vi "Launcher_Wheel_v4.vi"() -> ()   [LabVIEW 2011]
uses:
  StateMachineType.ctl
  BasketType.ctl
  FormulaChoose.ctl
  Robot Global Data.vi
  <vilib>/addons/control/pid/pid.llb/PID (DBL).vi
  <vilib>/addons/control/pid/NI_PID_pid.lvlib
panel:
  out "Encoder R":dbl
  out "Encoder L":dbl
  in  "PID R":T1={"proportional gain (Kc)"=0.0008, "integral time (Ti, min)"=0.010000000000000009, "derivative time (Td, min)"=0.0} {"derivative time (Td, min)" step=0.01 format="%.2f"; "integral time (Ti, min)" step=0.01 format="%.2f"; "proportional gain (Kc)" step=0.0001 format="%.4f"}
  in  "Output R":cluster{"output high":dbl, "output low":dbl}={"output high"=1.0, "output low"=0.0} {"output low" step=0.1 format="%.2f"; "output high" step=0.1 format="%.2f"}
  in  "Output L":cluster{"output high":dbl, "output low":dbl}={"output high"=1.0, "output low"=0.0} {"output low" step=0.1 format="%.2f"; "output high" step=0.1 format="%.2f"}
  in  "PID L":T1={"proportional gain (Kc)"=0.0008, "integral time (Ti, min)"=0.01, "derivative time (Td, min)"=0.0} {"derivative time (Td, min)" step=0.01 format="%.2f"; "integral time (Ti, min)" step=0.01 format="%.2f"; "proportional gain (Kc)" step=0.0001 format="%.4f"}
  out "R Status":bool
  out "L Status":bool
  in  "Encoder Control L (PC)":dbl(slide) step=100.0 scale=0.0..1400.0
  in  "Encoder Control R (PC)":dbl(slide) step=100.0 scale=0.0..1400.0
  in  "Set RPM (PC)":dbl(slide) step=100.0 scale=0.0..1400.0
  in  "Gamepad Adjust (PC)":dbl(slide) step=0.1 scale=1.0..-1.0
  in  "Autonomous (PC)":bool
  in  "Which Formula?":T2
  in  "Basket (PC)":T3=enum."Top"
  in  "Direct Motor Control":bool
  out "Calculation Failed":bool
  in  "Distance (PC)":dbl
  out "Motor R Input":dbl
  out "Motor L Input":dbl
  out "Loop Status":T4
  in  "RunLauncher (PC)":bool
  # "For testing on computer only"
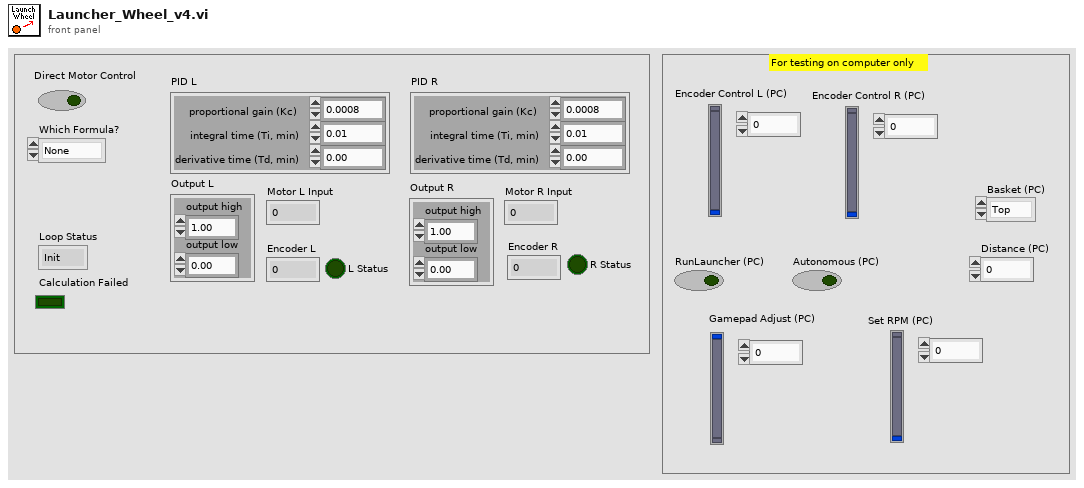
[diagram p1: front panel]
types:
  T1 = cluster{"proportional gain (Kc)":dbl, "integral time (Ti, min)":dbl, "derivative time (Td, min)":dbl}
  T2 = typedef "FormulaChoose.ctl" = enum16{"None", "Brian", "Jeremy", "Steven", "Data Based"}
  T3 = typedef "BasketType.ctl" = enum16{"Left", "Bottom", "Right", "Top"}
  T4 = typedef "StateMachineType.ctl" = enum16{"Init", "Idle", "Start", "Do", "Stop"}
  T5 = typedef "WPI_MotorControlDeviceRef.ctl" = cluster{"DeviceStatus":errorcluster, "Type":enum16{"PWM", "CAN"}, "PWM":cluster{"Digital Module":T6, "PWM Channel":T7, "DeadBand":T8}, "CAN":cluster{"Device Number":u8, "Control Mode":T9, "Semaphore":T10, "Max Vout":dbl}, "Invert":bool, "TransformRef":T11, "InvTransformRef":T11}
  T6 = typedef "FPGA_TypedefDigitalModule.ctl" = enum16{"Digital Module 1", "Digital Module 2"}
  T7 = typedef "FPGA_DIOPWMChannel.ctl" = enum8{"PWM 1", "PWM 2", "PWM 3", "PWM 4", "PWM 5", "PWM 6", "PWM 7", "PWM 8", "PWM 9", "PWM 10", "Invalid"}
  T8 = typedef "WPI_PWMDeadband.ctl" = cluster{"Name":string, "maxPositivePwm":i32, "minPositivePwm":i32, "centerPwm":i32, "maxNegativePwm":i32, "minNegativePwm":i32, "angularRange":u16}
  T9 = typedef "WPI_CANJaguar_ControlMode.ctl" = enum8{"Percent VBus", "Current", "Speed", "Position", "Voltage"}
  T10 = typedef "Semaphore RefNum" = refnum<k1>
  T11 = typedef "WPI_PWMTransform_ConPane.ctl" = refnum<vi>
  T12 = typedef "WPI_CounterDevRef.ctl" = cluster{"DevStatus":errorcluster, "CntIndex":T13}
  T13 = typedef "FPGA_CounterCtrSystemIndex.ctl" = enum8{"Ctr 0", "Ctr 1", "Ctr 2", "Ctr 3", "Ctr 4", "Ctr 5", "Ctr 6", "Ctr 7", "Invalid"}
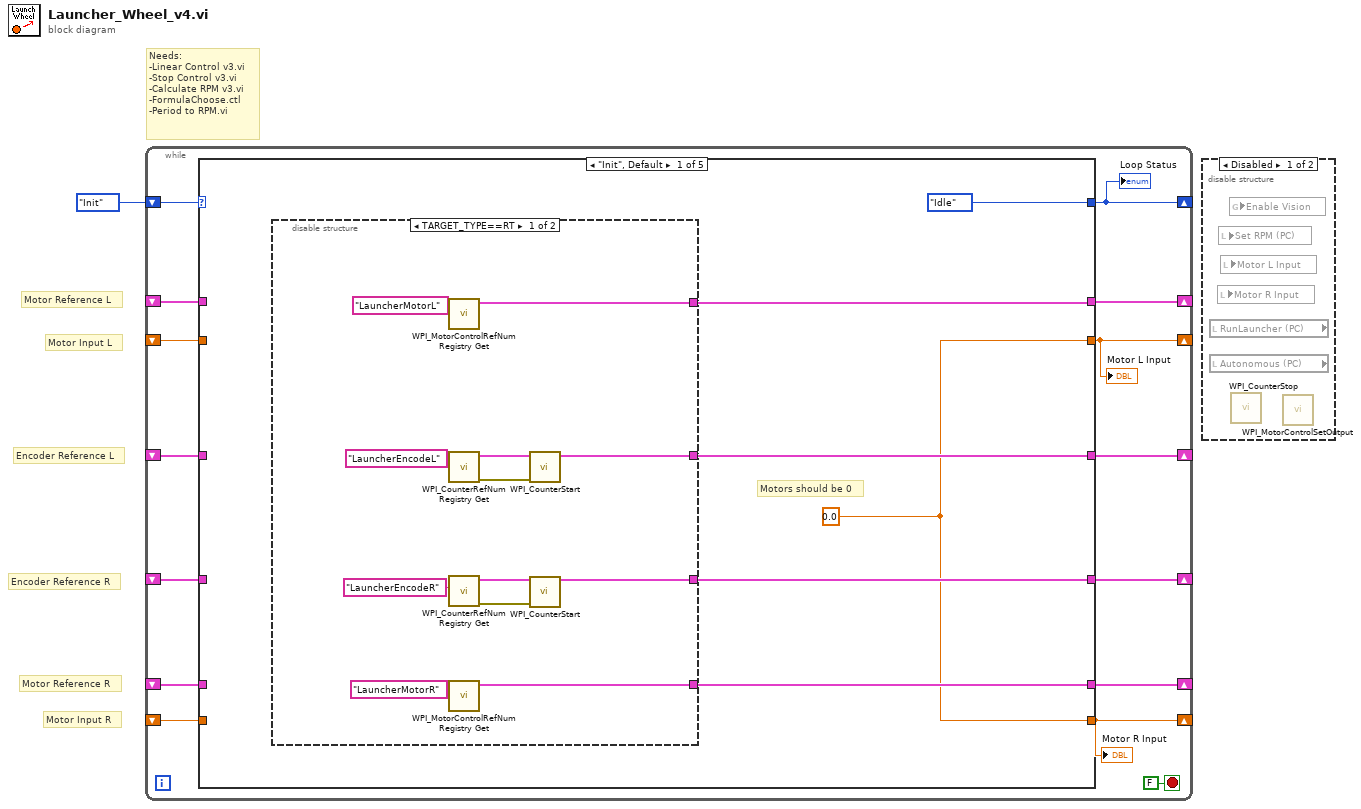
[diagram p0: block diagram]
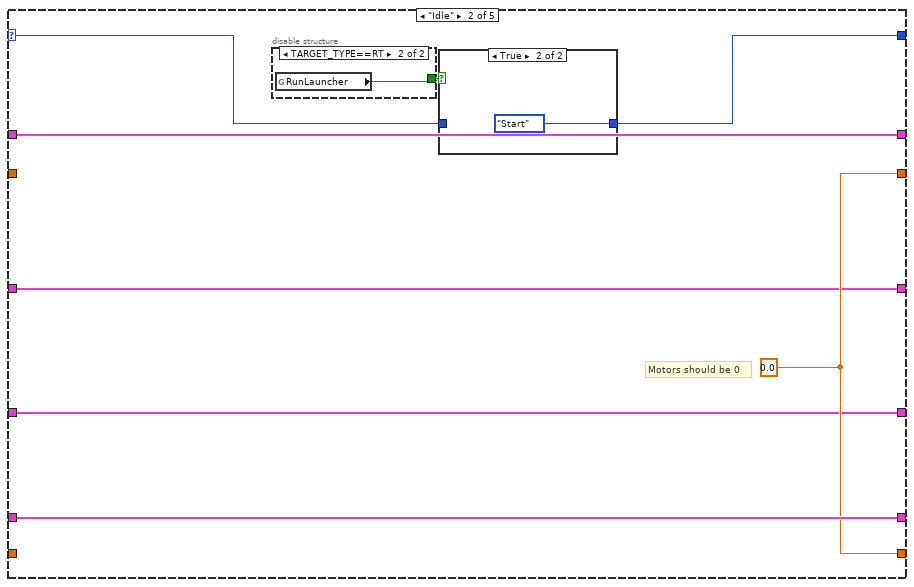
[diagram p4: hidden frame]
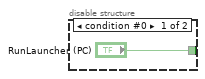
[diagram p5: hidden frame]
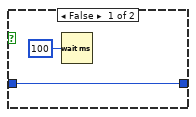
[diagram p6: hidden frame]
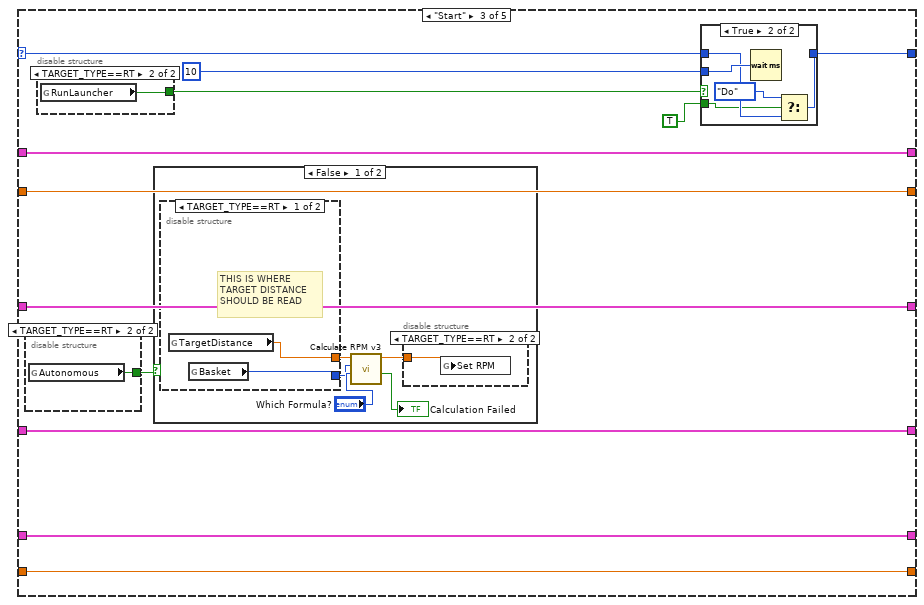
[diagram p7: hidden frame]
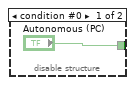
[diagram p8: hidden frame]
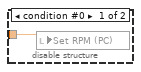
[diagram p9: hidden frame]
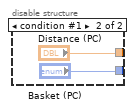
[diagram p10: hidden frame]
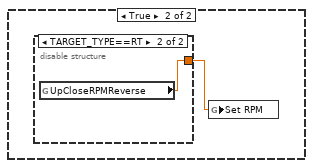
[diagram p11: hidden frame]
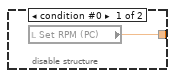
[diagram p12: hidden frame]
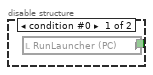
[diagram p13: hidden frame]
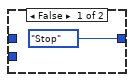
[diagram p14: hidden frame]
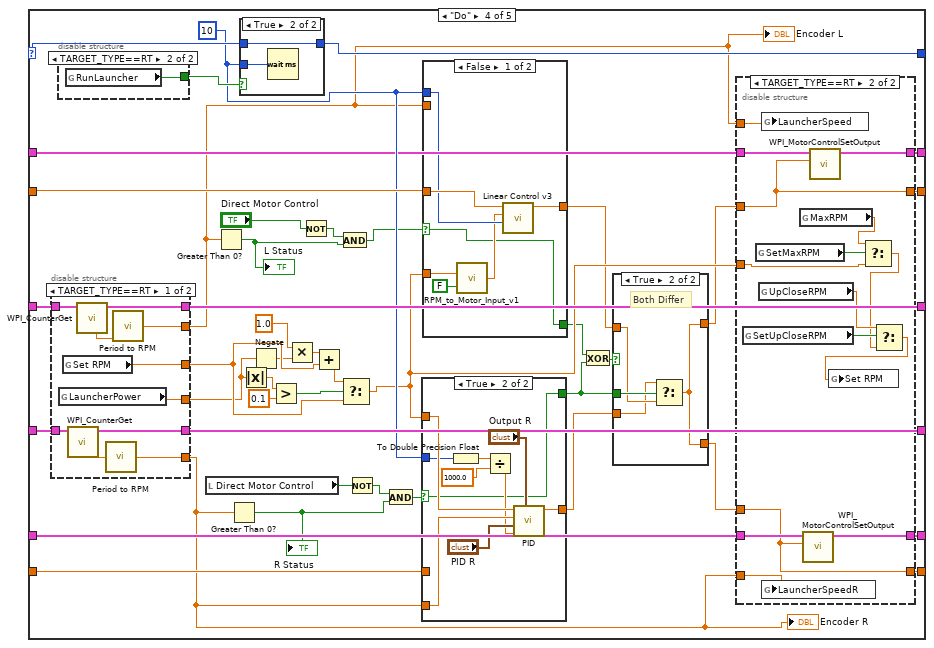
[diagram p15: hidden frame]
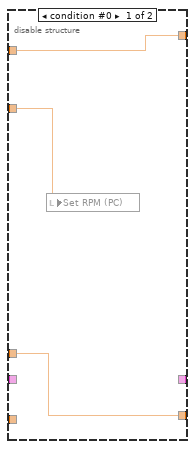
[diagram p17: hidden frame]
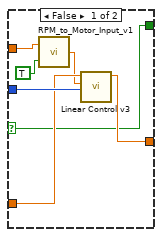
[diagram p18: hidden frame]
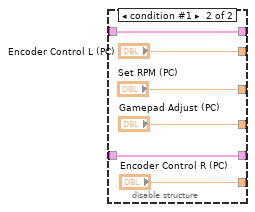
[diagram p19: hidden frame]
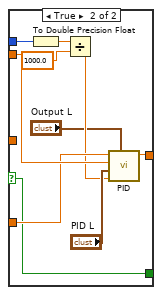
[diagram p20: hidden frame]
diagram:
  # "Needs:\n-Linear Control v3.vi\n-Stop Control v3.vi\n-Calculate RPM v3.vi\n-FormulaChoose.ctl\n-Period to RPM.vi"
  # "Motor Input R"
  # "Encoder Reference R"
  # "Motor Reference R"
  # "Encoder Reference L"
  # "Motor Reference L"
  # "Motor Input L"
  n1 = while {
    shift-right: [w2] -> _
    shift-left: StateMachineType."Init" ("Enum") -> [w15]
    shift-right: [w13] -> _
    shift-left: _ -> [w11]
    shift-right: [w14] -> _
    shift-left: _ -> [w12]
    shift-right: [w3] -> _
    shift-left: _ -> [w9]
    shift-right: [w4] -> _
    shift-left: _ -> [w10]
    shift-right: [w8] -> _
    shift-left: _ -> [w6]
    shift-right: [w7] -> _
    shift-left: _ -> [w5]
    stop <- FALSE stop-if-true
    n2 = case shown="\"Init\", Default" w15 {
      selector: w15 -> [_ w36 w57 w125 w215]
      tunnel: [StateMachineType."Idle" ("Enum") w35 w53 w124 w216] -> w2
      tunnel: [w21 w42 w51 w112 w214] -> w14
      tunnel: [w18 w41 w50 w111 w213] -> w13
      tunnel: w12 -> [_ w42 w51 w114 w211]
      tunnel: w11 -> [_ w41 w50 w113 w212]
      tunnel: [w17 w39 w48 w110 w209] -> w3
      tunnel: [w17 w39 w49 w109 w210] -> w4
      tunnel: w10 -> [_ _ w49 w117 w221]
      tunnel: w9 -> [_ _ w48 w116 w220]
      tunnel: [w19 w38 w56 w121 w208] -> w8
      tunnel: [w20 w37 w55 w120 w207] -> w7
      tunnel: w6 -> [_ w38 w56 w123 w208]
      tunnel: w5 -> [_ w37 w55 w122 w207]
      frame "Init", Default {
        w17 = 0.0
        # "Motors should be 0"
        n3 = disable-structure shown="TARGET_TYPE==RT" {
          disable-tunnel: [w32 _] -> w21
          disable-tunnel: [w31 _] -> w18
          disable-tunnel: [w27 _] -> w19
          disable-tunnel: [w28 _] -> w20
          frame condition #0 (active) {
            n4 = call <vilib>:"WPI_MotorControlRefNum Registry Get.vi"("refnum name"="LauncherMotorL") -> ("MotorControlDevRef"=w32:T5)  [unwired: 9 in, 1 out]
            n5 = call <vilib>:"WPI_CounterRefNum Registry Get.vi"("refnum name"="LauncherEncodeL") -> ("error out"=w23:errorcluster, "CounterDevRef"=w26:T12)  [unwired: 9 in]
            n6 = call <vilib>:"WPI_CounterRefNum Registry Get.vi"("refnum name"="LauncherEncodeR") -> ("error out"=w24:errorcluster, "CounterDevRef"=w25:T12)  [unwired: 9 in]
            n7 = call <vilib>:"WPI_MotorControlRefNum Registry Get.vi"("refnum name"="LauncherMotorR") -> ("MotorControlDevRef"=w31:T5)  [unwired: 9 in, 1 out]
            n8 = call <vilib>:"WPI_CounterStart.vi"("error in (no error)"=w23, "CounterDevRef in"=w26) -> ("CounterDevRef out"=w27:T12)  [unwired: 8 in, 1 out]
            n9 = call <vilib>:"WPI_CounterStart.vi"("error in (no error)"=w24, "CounterDevRef in"=w25) -> ("CounterDevRef out"=w28:T12)  [unwired: 8 in, 1 out]
          }
          frame condition #1 {
          }
        }
      }
      frame "Idle" {
        w39 = 0.0 ("New Motor Input")
        # "Motors should be 0"
        n10 = disable-structure shown="TARGET_TYPE==RT" {
          disable-tunnel: ["RunLauncher (PC)" w44] -> w40
          frame condition #0 {
          }
          frame condition #1 (active) {
            n11 = global read "Robot Global Data.vi" "RunLauncher"() -> (w44:bool)
          }
        }
        n12 = case shown="True" w40 {
          tunnel: w36 -> [w45 _]
          tunnel: [w45 StateMachineType."Start" ("Enum")] -> w35
          frame False {
            n13 = Wait (ms)(milliseconds to wait=u32 100) -> ()  [unwired: 1 out]
          }
          frame True {
          }
        }
      }
      frame "Start" {
        n14 = disable-structure shown="TARGET_TYPE==RT" {
          disable-tunnel: ["Autonomous (PC)" w61] -> w54
          frame condition #0 {
          }
          frame condition #1 (active) {
            n15 = global read "Robot Global Data.vi" "Autonomous"() -> (w61:bool)
          }
        }
        n16 = disable-structure shown="TARGET_TYPE==RT" {
          disable-tunnel: [w76 w77] -> w58
          frame condition #0 {
            n17 = local read "RunLauncher (PC)"() -> (w76:bool)
          }
          frame condition #1 (active) {
            n18 = global read "Robot Global Data.vi" "RunLauncher"() -> (w77:bool)
          }
        }
        n19 = case shown="False" w54 {
          frame False {
            n20 = disable-structure shown="TARGET_TYPE==RT" {
              disable-tunnel: [w69 "Distance (PC)"] -> w63
              disable-tunnel: [w70 "Basket (PC)"] -> w62
              frame condition #0 (active) {
                # "THIS IS WHERE\nTARGET DISTANCE\nSHOULD BE READ"
                n21 = global read "Robot Global Data.vi" "TargetDistance"() -> (w69:dbl)
                n22 = global read "Robot Global Data.vi" "Basket"() -> (w70:T3)
              }
              frame condition #1 {
              }
            }
            n23 = call "Calculate RPM v3.vi"("Which Formula"="Which Formula?", "Basket"=w62, "Distance to Target (feet)"=w63) -> ("Calculation Failed"=→"Calculation Failed":bool, "RPM"=w64:dbl)  [unwired: 6 in, 1 out]
            n24 = disable-structure shown="TARGET_TYPE==RT" {
              disable-tunnel: w64 -> [w67 w68]
              frame condition #0 {
                n25 = local write "Set RPM (PC)"(w67) -> ()
              }
              frame condition #1 (active) {
                n26 = global write "Robot Global Data.vi" "Set RPM"(w68) -> ()
              }
            }
          }
          frame True {
            n27 = disable-structure shown="TARGET_TYPE==RT" {
              disable-tunnel: [w74 w75] -> w73
              frame condition #0 {
                n28 = local read "Set RPM (PC)"() -> (w74:dbl)
              }
              frame condition #1 (active) {
                n29 = global read "Robot Global Data.vi" "UpCloseRPMReverse"() -> (w75:dbl)
              }
            }
            n30 = global write "Robot Global Data.vi" "Set RPM"(w73) -> ()
          }
        }
        n31 = case shown="True" w58 {
          tunnel: u32 10 ("milliseconds to wait") -> [_ w83]
          tunnel: [StateMachineType."Stop" w80] -> w53
          tunnel: w57 -> [_ w82]
          tunnel: TRUE -> [_ w79]
          frame False {
          }
          frame True {
            n32 = Wait (ms)(milliseconds to wait=w83) -> ()  [unwired: 1 out]
            n33 = Select(t=StateMachineType."Do" ("Enum"), s=w79, f=w82) -> (s? t:f=w80:T4)
          }
        }
      }
      frame "Do" {
        w115 = u32 10 ("milliseconds to wait")
        n34 = disable-structure shown="TARGET_TYPE==RT" {
          disable-tunnel: w122 -> [w168 w182]
          disable-tunnel: w123 -> [w177 w183]
          disable-tunnel: [w176 w182] -> w120
          disable-tunnel: [w175 w183] -> w121
          disable-tunnel: [w171 "Encoder Control L (PC)"] -> w107
          disable-tunnel: [w173 "Encoder Control R (PC)"] -> w108
          disable-tunnel: [w170 "Set RPM (PC)"] -> w119
          disable-tunnel: [w169 "Gamepad Adjust (PC)"] -> w118
          frame condition #0 (active) {
            n35 = global read "Robot Global Data.vi" "LauncherPower"() -> (w169:dbl)
            n36 = global read "Robot Global Data.vi" "Set RPM"() -> (w170:dbl)
            n37 = call <vilib>:"WPI_CounterGet.vi"("CounterDevRef in"=w168) -> ("CounterDevRef out"=w176:T12, "Period (sec)"=w174:dbl)  [unwired: 5 in, 4 out]
            n38 = call <vilib>:"WPI_CounterGet.vi"("CounterDevRef in"=w177) -> ("CounterDevRef out"=w175:T12, "Period (sec)"=w172:dbl)  [unwired: 5 in, 4 out]
            n39 = call "Period to RPM.vi"("Period (sec)"=w174) -> ("Numeric Control"=w173:dbl)
            n40 = call "Period to RPM.vi"("Period (sec)"=w172) -> ("Numeric Control"=w171:dbl)
          }
          frame condition #1 {
          }
        }
        "Encoder R" <- w108
        "Encoder L" <- w107
        n41 = disable-structure shown="TARGET_TYPE==RT" {
          disable-tunnel: [w201 w202] -> w126
          frame condition #0 {
            n42 = local read "RunLauncher (PC)"() -> (w201:bool)
          }
          frame condition #1 (active) {
            n43 = global read "Robot Global Data.vi" "RunLauncher"() -> (w202:bool)
          }
        }
        n44 = local read "Direct Motor Control"() -> (w98:bool)
        n45 = Greater Than 0?(x=w107) -> (x > 0?=w93:bool)
        "L Status" <- w93
        n46 = Greater Than 0?(x=w108) -> (x > 0?=w96:bool)
        "R Status" <- w96
        n47 = case shown="True" w126 {
          tunnel: w115 -> [_ w205]
          tunnel: w125 -> [_ w204]
          tunnel: [StateMachineType."Stop" ("Enum") w204] -> w124
          frame False {
          }
          frame True {
            n48 = Wait (ms)(milliseconds to wait=w205) -> ()  [unwired: 1 out]
          }
        }
        n49 = Absolute Value(x=w118) -> (abs(x)=w104:dbl)
        n50 = Negate(x=w118) -> (-x=w103:dbl)
        n51 = Greater?(x=w104, y=0.1) -> (0:w105:bool)
        n52 = Multiply(x=1.0, y=w103) -> (x*y=w101:dbl)
        n53 = Not(x="Direct Motor Control") -> (.not. x?=w94:bool)
        n54 = Add(x=w101, y=w119) -> (x+y=w100:dbl)
        n55 = And(x=w94, y=w93) -> (x .and. y?=w91:bool)
        n56 = Select(t=w100, s=w105, f=w119) -> (s? t:f=w99:dbl)
        n57 = Not(x=w98) -> (.not. x?=w97:bool)
        n58 = And(x=w97, y=w96) -> (x .and. y?=w95:bool)
        n59 = case shown="True" w95 {
          selector: w95 -> [w151 w158]
          tunnel: w116 -> [w156 _]
          tunnel: w99 -> [w153 w165]
          tunnel: w108 -> [_ w164]
          tunnel: w115 -> [w157 w161]
          tunnel: [w155 w159] -> w86
          tunnel: [w151 w158] -> w88
          frame False {
            n60 = call "RPM_to_Motor_Input_v1.vi"("Right Motor?"=TRUE, "RPM"=w153) -> ("Motor Input"=w154:dbl)
            n61 = call "Linear Control v3.vi"("Loop Time (ms)"=w157, "Setpoint"=w154, "Recieved Motor Input"=w156) -> ("New Motor Input"=w155:dbl)  [unwired: 7 in, 1 out]
          }
          frame True {
            n62 = To Double Precision Float(number=w161) -> (double precision float=w163:dbl)
            n63 = Divide(x=w163, y=1000.0) -> (x/y=w160:dbl)
            n64 = call-poly <vilib>:"PID.vi"("output range"="Output R", "dt (s)"=w160, "PID gains"="PID R", "process variable"=w164, "setpoint"=w165) -> ("output"=w159:dbl)  [unwired: 5 in, 1 out]
          }
        }
        n65 = case shown="False" w91 {
          selector: w91 -> [w184 w191]
          tunnel: w117 -> [w190 _]
          tunnel: w99 -> [w186 w199]
          tunnel: w107 -> [_ w200]
          tunnel: w115 -> [w189 w197]
          tunnel: [w188 w192] -> w87
          tunnel: [w184 w191] -> w89
          frame False {
            n66 = call "RPM_to_Motor_Input_v1.vi"("Right Motor?"=FALSE, "RPM"=w186) -> ("Motor Input"=w187:dbl)
            n67 = call "Linear Control v3.vi"("Loop Time (ms)"=w189, "Setpoint"=w187, "Recieved Motor Input"=w190) -> ("New Motor Input"=w188:dbl)  [unwired: 7 in, 1 out]
          }
          frame True {
            n68 = To Double Precision Float(number=w197) -> (double precision float=w196:dbl)
            n69 = Divide(x=w196, y=1000.0) -> (x/y=w194:dbl)
            n70 = call-poly <vilib>:"PID.vi"("output range"="Output L", "dt (s)"=w194, "PID gains"="PID L", "process variable"=w200, "setpoint"=w199) -> ("output"=w192:dbl)  [unwired: 5 in, 1 out]
          }
        }
        n71 = Exclusive Or(1:w88, 2:w89) -> (0:w90:bool)
        n72 = case shown="True" w90 {
          tunnel: w88 -> [_ w132]
          tunnel: w87 -> [w128 w131]
          tunnel: w86 -> [w127 w130]
          tunnel: [w128 w129] -> w85
          tunnel: [w127 w129] -> w84
          frame False {
            # "Both Same"
          }
          frame True {
            # "Both Differ"
            n73 = Select(t=w130, s=w132, f=w131) -> (s? t:f=w129:dbl)
          }
        }
        n74 = disable-structure shown="TARGET_TYPE==RT" {
          disable-tunnel: w114 -> [_ w150]
          disable-tunnel: w113 -> [_ w148]
          disable-tunnel: w85 -> [w135 w145]
          disable-tunnel: w84 -> [w134 w146]
          disable-tunnel: [_ w149] -> w112
          disable-tunnel: [_ w147] -> w111
          disable-tunnel: [w134 w146] -> w110
          disable-tunnel: [w135 w145] -> w109
          disable-tunnel: w99 -> [w133 w138]
          disable-tunnel: w107 -> [_ w144]
          disable-tunnel: w108 -> [_ w143]
          frame condition #0 {
            n75 = local write "Set RPM (PC)"(w133) -> ()
          }
          frame condition #1 (active) {
            n76 = global read "Robot Global Data.vi" "SetUpCloseRPM"() -> (w142:bool)
            n77 = global read "Robot Global Data.vi" "SetMaxRPM"() -> (w139:bool)
            n78 = global read "Robot Global Data.vi" "UpCloseRPM"() -> (w140:dbl)
            n79 = global write "Robot Global Data.vi" "LauncherSpeed"(w144) -> ()
            n80 = global write "Robot Global Data.vi" "LauncherSpeedR"(w143) -> ()
            n81 = global read "Robot Global Data.vi" "MaxRPM"() -> (w137:dbl)
            n82 = call <vilib>:"WPI_MotorControlSetOutput.vi"("Output"=w146, "MotorControlDevRef"=w148) -> ("MotorControlDevRef"=w147:T5)  [unwired: 8 in, 1 out]
            n83 = call <vilib>:"WPI_MotorControlSetOutput.vi"("Output"=w145, "MotorControlDevRef"=w150) -> ("MotorControlDevRef"=w149:T5)  [unwired: 8 in, 1 out]
            n84 = Select(t=w137, s=w139, f=w138) -> (s? t:f=w136:dbl)
            n85 = Select(t=w140, s=w142, f=w136) -> (s? t:f=w141:dbl)
            n86 = global write "Robot Global Data.vi" "Set RPM"(w141) -> ()
          }
        }
      }
      frame "Stop" {
        w206 = 0.5 ("Rate (unit/s)")
        w219 = u32 10 ("milliseconds to wait")
        n87 = disable-structure shown="TARGET_TYPE==RT" {
          disable-tunnel: [w224 w225] -> w218
          frame condition #0 {
            n88 = local read "RunLauncher (PC)"() -> (w224:bool)
          }
          frame condition #1 (active) {
            n89 = global read "Robot Global Data.vi" "RunLauncher"() -> (w225:bool)
          }
        }
        n90 = call "Stop Control v3.vi"("Rate (unit/s)"=w206, "Loop Time (ms)"=w219, "Recieved Motor Input"=w221) -> ("Done Stopping"=w222:bool, "New Motor Input"=w210:dbl)  [unwired: 7 in]
        n91 = call "Stop Control v3.vi"("Rate (unit/s)"=w206, "Loop Time (ms)"=w219, "Recieved Motor Input"=w220) -> ("Done Stopping"=w223:bool, "New Motor Input"=w209:dbl)  [unwired: 7 in]
        n92 = And(x=w222, y=w223) -> (x .and. y?=w217:bool)
        n93 = case shown="False" w218 {
          tunnel: w219 -> [w236 _]
          tunnel: w217 -> [w233 _]
          tunnel: [w234 StateMachineType."Start" ("Enum")] -> w216
          tunnel: w215 -> [w232 _]
          frame False {
            n94 = Wait (ms)(milliseconds to wait=w236) -> ()  [unwired: 1 out]
            n95 = Select(t=StateMachineType."Idle" ("Enum"), s=w233, f=w232) -> (s? t:f=w234:T4)
          }
          frame True {
          }
        }
        n96 = disable-structure shown="TARGET_TYPE==RT" {
          disable-tunnel: [w231 _] -> w214
          disable-tunnel: [w230 _] -> w213
          disable-tunnel: w212 -> [w229 _]
          disable-tunnel: w211 -> [w228 _]
          disable-tunnel: w210 -> [w227 _]
          disable-tunnel: w209 -> [w226 _]
          frame condition #0 (active) {
            n97 = call <vilib>:"WPI_MotorControlSetOutput.vi"("Output"=w227, "MotorControlDevRef"=w228) -> ("MotorControlDevRef"=w231:T5)  [unwired: 8 in, 1 out]
            n98 = call <vilib>:"WPI_MotorControlSetOutput.vi"("Output"=w226, "MotorControlDevRef"=w229) -> ("MotorControlDevRef"=w230:T5)  [unwired: 8 in, 1 out]
          }
          frame condition #1 {
          }
        }
      }
    }
    "Loop Status" <- w2
    "Motor R Input" <- w3
    "Motor L Input" <- w4
  }
  n99 = disable-structure shown="Disabled" {
    frame Disabled {
      n100 = local read "RunLauncher (PC)"() -> ()  [unwired: 1 out]
      n101 = local read "Autonomous (PC)"() -> ()  [unwired: 1 out]
      n102 = local read "Motor R Input"() -> ()  [unwired: 1 in]
      n103 = local read "Set RPM (PC)"() -> ()  [unwired: 1 in]
      n104 = local read "Motor L Input"() -> ()  [unwired: 1 in]
      n105 = global read "Robot Global Data.vi" "Enable Vision"() -> ()  [unwired: 1 in]
      n106 = call <vilib>:"WPI_CounterStop.vi"() -> ()  [unwired: 10 in, 2 out]
      n107 = call <vilib>:"WPI_MotorControlSetOutput.vi"() -> ()  [unwired: 10 in, 2 out]
    }
    frame Enabled {
    }
  }
